vi "Begin.vi"(11 "Image Size":T1=enum."160x120") -> (0 "error out":errorcluster)   [LabVIEW 2012]
doc: "Called before other user functions, this VI is expected to open initial I/O refnums, load in file data, and do all program initialization. Notice that the <B>error out</B> terminal is simply used for data flow. Wiring it to other structures or subVIs ensures that this VI runs first."
uses:
  <vilib>/Rock Robotics/WPI/Camera/WPI_CameraImageSize.ctl
  <vilib>/Rock Robotics/SystemInterfaces/DIO/FPGA_DIOPWMChannel.ctl
  <vilib>/Rock Robotics/WPI/Camera/WPI_CameraWhite Balance Values.ctl
  <vilib>/Rock Robotics/WPI/Camera/WPI_CameraExposure Values.ctl
  <vilib>/Rock Robotics/WPI/Camera/WPI_CameraFrameRate.ctl
  <vilib>/Rock Robotics/WPI/DriverStation/WPI_DriverStationRobotMode2.ctl
  <vilib>/Rock Robotics/WPI/Joystick/WPI_JoystickDeviceEnum.ctl
  <vilib>/Rock Robotics/WPI/SafetyOutput/WPI_SafetyOutputConfigMenu.ctl
  <vilib>/Rock Robotics/SystemInterfaces/DIO/FPGA_DIOChannel.ctl
  <vilib>/Rock Robotics/SystemInterfaces/DIO/FPGA_DIORelayChannel.ctl
  <vilib>/Rock Robotics/WPI/Solenoid/WPI_SolenoidChannel.ctl
  <vilib>/Rock Robotics/SystemInterfaces/Typedef/FPGA_TypedefSolenoidModule.ctl
  <vilib>/Rock Robotics/SystemInterfaces/Typedef/FPGA_TypedefDigitalModule.ctl
  <vilib>/Rock Robotics/SystemInterfaces/Typedef/FPGA_TypedefAnalogModuleForGyro.ctl
  <vilib>/Rock Robotics/SystemInterfaces/AI/FPGA_AIGyroChannel.ctl
  <vilib>/Rock Robotics/WPI/RobotDrive/WPI_RobotDriveOpen2MotorWithJaguar.vi
  Robot Global Data.vi
  <vilib>/Rock Robotics/WPI/RobotDrive/WPI_RobotDriveOpen2MotorWithVictor.vi
  <vilib>/Rock Robotics/WPI/Solenoid/WPI_SolenoidOpenDouble.vi
  <vilib>/Rock Robotics/WPI/Compressor/WPI_CompressorGetSetRefNum.vi
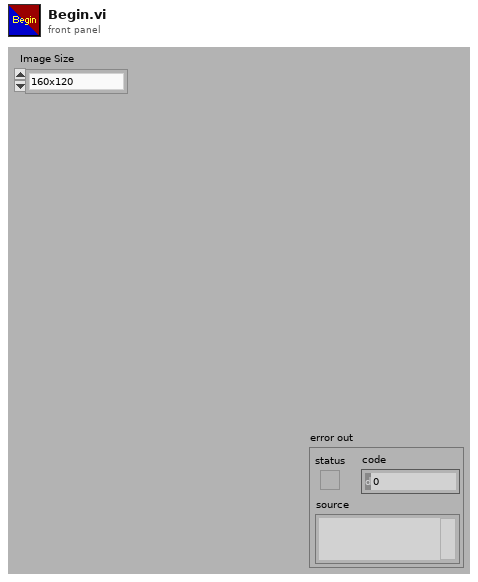
[diagram p1: front panel]
types:
  T1 = typedef "WPI_CameraImageSize.ctl" = enum16{"640x480", "320x240", "160x120"}
  T2 = typedef "FPGA_AIGyroChannel.ctl" = enum8{"AI 1", "AI 2", "Invalid"}
  T3 = typedef "FPGA_TypedefAnalogModuleForGyro.ctl" = enum16{"Analog Module 1"}
  T4 = typedef "FPGA_TypedefDigitalModule.ctl" = enum16{"Digital Module 1", "Digital Module 2"}
  T5 = typedef "WPI_SolenoidChannel.ctl" = enum8{"Solenoid 1", "Solenoid 2", "Solenoid 3", "Solenoid 4", "Solenoid 5", "Solenoid 6", "Solenoid 7", "Solenoid 8", "Invalid"}
  T6 = typedef "FPGA_TypedefSolenoidModule.ctl" = enum16{"Solenoid Module 1", "Solenoid Module 2"}
  T7 = typedef "FPGA_DIORelayChannel.ctl" = enum8{"Relay 1", "Relay 2", "Relay 3", "Relay 4", "Relay 5", "Relay 6", "Relay 7", "Relay 8", "Invalid"}
  T8 = typedef "FPGA_DIOChannel.ctl" = enum8{"DIO 1", "DIO 2", "DIO 3", "DIO 4", "DIO 5", "DIO 6", "DIO 7", "DIO 8", "DIO 9", "DIO 10", "DIO 11", "DIO 12", "DIO 13", "DIO 14", "Invalid"}
  T9 = typedef "WPI_SafetyOutputConfigMenu.ctl" = enum16{"Enable", "Disable"}
  T10 = typedef "FPGA_DIOPWMChannel.ctl" = enum8{"PWM 1", "PWM 2", "PWM 3", "PWM 4", "PWM 5", "PWM 6", "PWM 7", "PWM 8", "PWM 9", "PWM 10", "Invalid"}
  T11 = typedef "WPI_JoystickDeviceEnum.ctl" = enum16{"USB 1", "USB 2", "USB 3", "USB 4", "Kinect 1", "Kinect 2"}
  T12 = typedef "WPI_DriverStationRobotMode2.ctl" = enum16{"Autonomous Disabled", "Autonomous Enabled", "Teleop Disabled", "Teleop Enabled", "Timeout", "Finish", "Test Disabled", "Test Enabled"}
  T13 = typedef "WPI_CameraFrameRate.ctl" = u32
  T14 = typedef "WPI_CameraExposure Values.ctl" = enum16{"Auto", "Flicker-free 50 Hz", "Flicker-free 60 Hz", "Hold current"}
  T15 = typedef "WPI_CameraWhite Balance Values.ctl" = enum16{"Auto", "Fixed indoor", "Fixed outdoor 1", "Fixed outdoor 2", "Fixed fluorescent 1", "Fixed fluorescent 2", "Hold current"}
  T16 = typedef "WPI_CameraDevRef.ctl" = cluster{"Camera Address":string, "CameraStatus":errorcluster, "Acquire Image Notifier":refnum<notifier>}
  T17 = typedef "WPI_JoystickDevRef.ctl" = cluster{"Device":T11}
  T18 = typedef "WPI_RobotDriveDevRef.ctl" = cluster{"DevStatus":errorcluster, "Motors[]":T19[], "Square Inputs":bool, "Max Output":dbl, "Isochronous":bool}
  T19 = typedef "WPI_MotorControlDeviceRef.ctl" = cluster{"DeviceStatus":errorcluster, "Type":enum16{"PWM", "CAN"}, "PWM":cluster{"Digital Module":T4, "PWM Channel":T10, "DeadBand":T20}, "CAN":cluster{"Device Number":u8, "Control Mode":T21, "Semaphore":T22, "Max Vout":dbl}, "Invert":bool, "TransformRef":T23, "InvTransformRef":T23}
  T20 = typedef "WPI_PWMDeadband.ctl" = cluster{"Name":string, "maxPositivePwm":i32, "minPositivePwm":i32, "centerPwm":i32, "maxNegativePwm":i32, "minNegativePwm":i32, "angularRange":u16}
  T21 = typedef "WPI_CANJaguar_ControlMode.ctl" = enum8{"Percent VBus", "Current", "Speed", "Position", "Voltage"}
  T22 = typedef "Semaphore RefNum" = refnum<k1>
  T23 = typedef "WPI_PWMTransform_ConPane.ctl" = refnum<vi>
  T24 = typedef "WPI_CompressorDevRef.ctl" = cluster{"DevStatus":errorcluster, "DigitalInputDevRef":T25, "RelayDevRef":T26}
  T25 = typedef "WPI_DigitalInputDevRef.ctl" = cluster{"DevStatus":errorcluster, "DIO Channel":T8, "Digital Module":T4}
  T26 = typedef "WPI_RelayDevRef.ctl" = cluster{"DevStatus":errorcluster, "Relay Channel":T7, "Digital Module":T4, "Relay Direction":T27}
  T27 = typedef "WPI_RelayDirection.ctl" = enum16{"Both directions", "Forward only", "Reverse only"}
  T28 = typedef "WPI_SolenoidDevRef.ctl" = cluster{"DevStatus":errorcluster, "Solenoid Module":T6, "Forward Solenoid Channel":T5, "Reverse Solenoid Channel":T5}
  T29 = typedef "WPI_GyroDevRef.ctl" = cluster{"DevStatus":errorcluster, "Analog Module":T30, "Analog Channel":T31, "Offset":dbl, "Gain (VoltsPerDegree/Second)":dbl}
  T30 = typedef "FPGA_TypedefAnalogModule.ctl" = enum16{"Analog Module 1", "Analog Module 2"}
  T31 = typedef "FPGA_AIChannel.ctl" = enum8{"AI 1", "AI 2", "AI 3", "AI 4", "AI 5", "AI 6", "AI 7", "AI 8", "Invalid"}
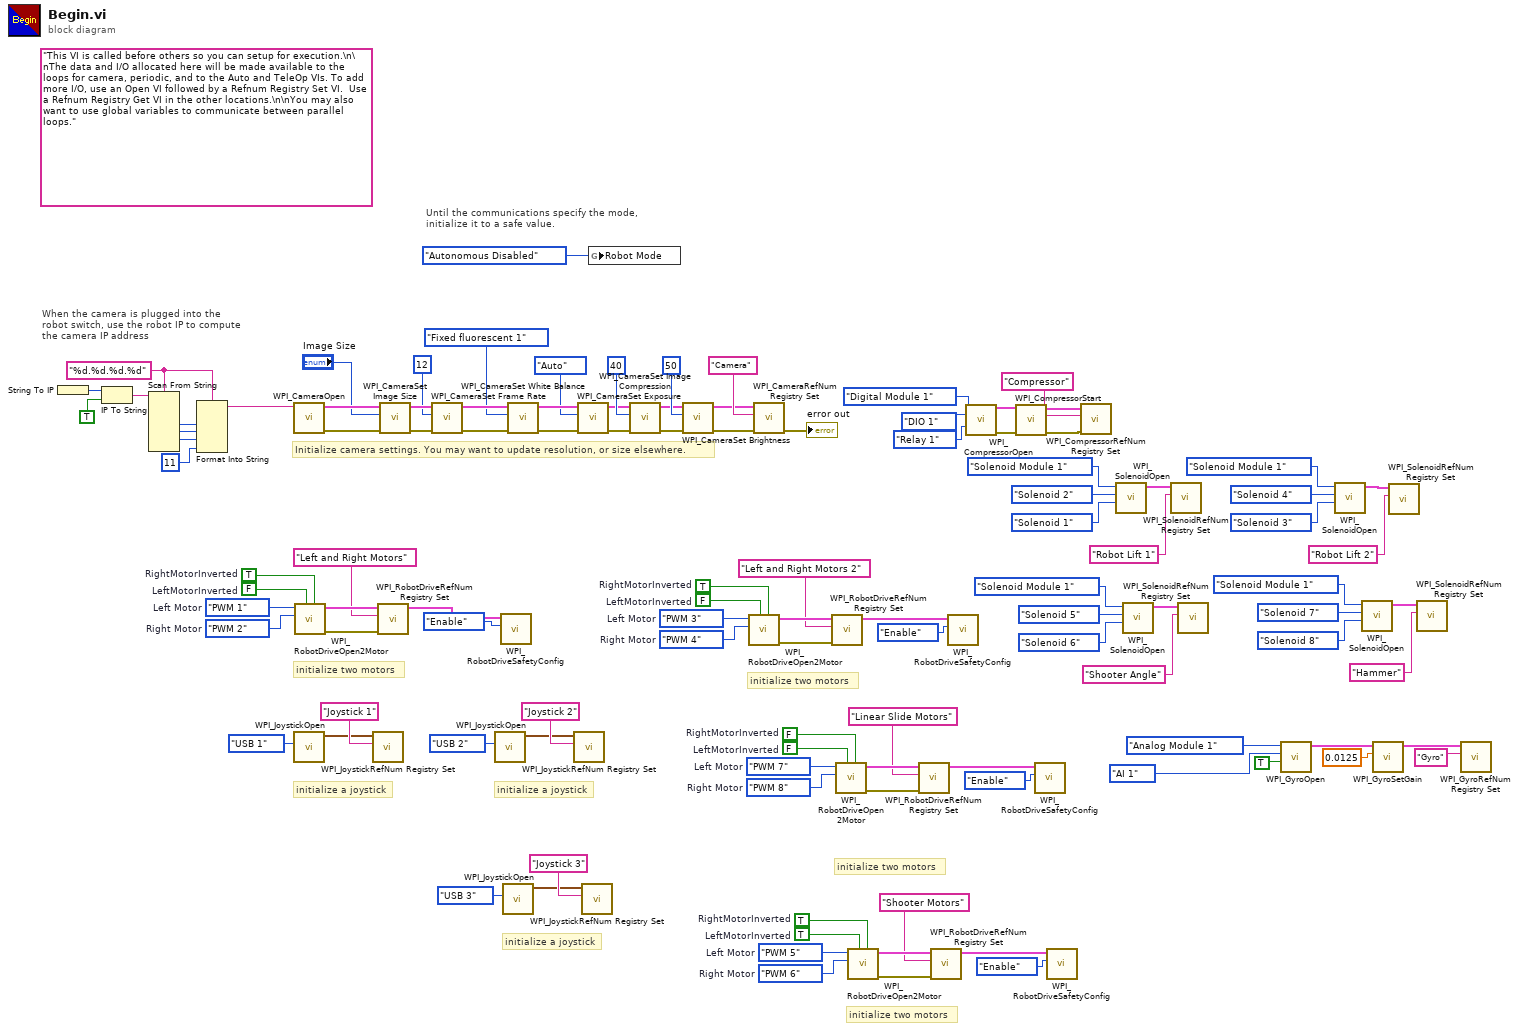
[diagram p0: block diagram]
diagram:
  w38 = FPGA_DIOPWMChannel."PWM 6"  # Right Motor
  w39 = FPGA_DIOPWMChannel."PWM 5"  # Left Motor
  w43 = TRUE  # LeftMotorInverted
  w44 = TRUE  # RightMotorInverted
  w50 = FPGA_DIOPWMChannel."PWM 8"  # Right Motor
  w51 = FPGA_DIOPWMChannel."PWM 7"  # Left Motor
  w55 = FALSE  # LeftMotorInverted
  w56 = FALSE  # RightMotorInverted
  w59 = FPGA_DIOPWMChannel."PWM 4"  # Right Motor
  w60 = FPGA_DIOPWMChannel."PWM 3"  # Left Motor
  w64 = FALSE  # LeftMotorInverted
  w65 = TRUE  # RightMotorInverted
  w77 = "%d.%d.%d.%d" ("format string")
  (unwired) "This VI is called before others so you can setup for execution.\n\nThe data and I/O allocated here will be made available to the loops for camera, periodic, and to the Auto and TeleOp VIs. To add more I/O, use an Open VI followed by a Refnum Registry Set VI.  Use a Refnum Registry Get VI in the other locations.\n\nYou may also want to use global variables to communicate between parallel loops."
  w88 = FPGA_DIOPWMChannel."PWM 2"  # Right Motor
  w89 = FPGA_DIOPWMChannel."PWM 1"  # Left Motor
  w111 = FALSE  # LeftMotorInverted
  w112 = TRUE  # RightMotorInverted
  # "initialize two motors"
  # "initialize a joystick"
  # "initialize two motors"
  # "initialize two motors"
  # "initialize a joystick"
  # "initialize a joystick"
  # "Until the communications specify the mode,\ninitialize it to a safe value."
  # "When the camera is plugged into the\nrobot switch, use the robot IP to compute\nthe camera IP address"
  # "initialize two motors"
  # "Initialize camera settings. You may want to update resolution, or size elsewhere."
  n1 = String To IP() -> (0:w84:u32)  [unwired: 1 in]
  n2 = IP To String(1:TRUE ("dot notation? (F)"), 2:w84) -> (0:w82:string)
  n3 = Scan From String(format string=w77, input string=w82) -> (output 1=w81:i32, output 2=w80:i32, output 3=w79:i32)  [unwired: 7 in, 3 out]
  n4 = Format Into String(format string=w77, w81, w80, w79, 11 ("Compression")) -> (resulting string=w73:string)  [unwired: 2 in, 1 out]
  n5 = call <vilib>:"WPI_CameraOpen.vi"("Camera Address"=w73) -> ("error out"=w98:errorcluster, "CameraDevRef"=w99:T16)  [unwired: 1 in, 8 out]
  n6 = call <vilib>:"WPI_JoystickOpen.vi"("JoystickDevice"=WPI_JoystickDeviceEnum."USB 1") -> ("JoystickDevRef"=w71:T17)  [unwired: 10 in]
  n7 = call-poly <vilib>:"WPI_RobotDriveOpen2Motor.vi"("Right Motor Inverted"=w112, "Left Motor Inverted"=w111, "Right Motor"=w88, "Left Motor"=w89) -> ("error out"=w107:errorcluster, "RobotDriveDevRef"=w109:T18)  [unwired: 1 in, 5 out]
  n8 = call <vilib>:"WPI_JoystickRefNum Registry Set.vi"("refnum name"="Joystick 1", "JoystickDevRef"=w71) -> ()  [unwired: 8 in, 2 out]
  n9 = call <vilib>:"WPI_RobotDriveRefNum Registry Set.vi"("error in (no error)"=w107, "refnum name"="Left and Right Motors", "RobotDriveDevRef"=w109) -> ("RobotDriveDevRef"=w76:T18)  [unwired: 8 out]
  n10 = call <vilib>:"WPI_CameraSet Image Size.vi"("error in (no error)"=w98, "Image Size"="Image Size", "CameraDevRef"=w99) -> ("error out"=w97:errorcluster, "CameraDevRef Out"=w100:T16)  [unwired: 7 out]
  n11 = call <vilib>:"WPI_CameraSet Frame Rate.vi"("error in (no error)"=w97, "Frame Rate (fps)"=T13 12, "CameraDevRef"=w100) -> ("error out"=w96:errorcluster, "CameraDevRef Out"=w102:T16)  [unwired: 7 out]
  n12 = call <vilib>:"WPI_JoystickOpen.vi"("JoystickDevice"=WPI_JoystickDeviceEnum."USB 2") -> ("JoystickDevRef"=w67:T17)  [unwired: 10 in]
  n13 = call <vilib>:"WPI_RobotDriveSafetyConfig.vi"("mode"=WPI_SafetyOutputConfigMenu."Enable", "RobotDriveDevRef"=w76) -> ()  [unwired: 8 in, 2 out]
  n14 = call <vilib>:"WPI_JoystickOpen.vi"("JoystickDevice"=WPI_JoystickDeviceEnum."USB 3") -> ("JoystickDevRef"=w46:T17)  [unwired: 10 in]
  n15 = call <vilib>:"WPI_CameraSet White Balance.vi"("error in (no error)"=w96, "White Balance"=WPI_CameraWhite_Balance_Values."Fixed fluorescent 1", "CameraDevRef"=w102) -> ("error out"=w95:errorcluster, "CameraDevRef Out"=w101:T16)  [unwired: 7 out]
  n16 = call <vilib>:"WPI_JoystickRefNum Registry Set.vi"("refnum name"="Joystick 2", "JoystickDevRef"=w67) -> ()  [unwired: 8 in, 2 out]
  n17 = call <vilib>:"WPI_CameraSet Exposure.vi"("error in (no error)"=w95, "Exposure"=WPI_CameraExposure_Values."Auto", "CameraDevRef"=w101) -> ("error out"=w94:errorcluster, "CameraDevRef Out"=w104:T16)  [unwired: 7 out]
  n18 = call <vilib>:"WPI_JoystickRefNum Registry Set.vi"("refnum name"="Joystick 3", "JoystickDevRef"=w46) -> ()  [unwired: 8 in, 2 out]
  n19 = global write "Robot Global Data.vi" "Robot Mode"(WPI_DriverStationRobotMode2."Autonomous Disabled" ("Robot Mode")) -> ()
  n20 = call <vilib>:"WPI_CameraSet Image Compression.vi"("error in (no error)"=w94, "Compression"=40, "CameraDevRef"=w104) -> ("error out"=w93:errorcluster, "CameraDevRef Out"=w103:T16)  [unwired: 7 out]
  n21 = call <vilib>:"WPI_CameraSet Brightness.vi"("error in (no error)"=w93, "Brightness"=50, "CameraDevRef"=w103) -> ("error out"=w91:errorcluster, "CameraDevRef Out"=w92:T16)  [unwired: 7 out]
  n22 = call-poly <vilib>:"WPI_RobotDriveOpen2Motor.vi"("Right Motor Inverted"=w65, "Left Motor Inverted"=w64, "Right Motor"=w59, "Left Motor"=w60) -> ("error out"=w61:errorcluster, "RobotDriveDevRef"=w63:T18)  [unwired: 1 in, 5 out]
  n23 = call <vilib>:"WPI_CameraRefNum Registry Set.vi"("error in (no error)"=w91, "refnum name"="Camera", "CameraDevRef"=w92) -> ("error out"=→"error out":errorcluster)  [unwired: 8 out]
  n24 = call <vilib>:"WPI_RobotDriveRefNum Registry Set.vi"("error in (no error)"=w61, "refnum name"="Left and Right Motors 2", "RobotDriveDevRef"=w63) -> ("RobotDriveDevRef"=w58:T18)  [unwired: 8 out]
  n25 = call-poly <vilib>:"WPI_RobotDriveOpen2Motor.vi"("Right Motor Inverted"=w56, "Left Motor Inverted"=w55, "Right Motor"=w50, "Left Motor"=w51) -> ("error out"=w52:errorcluster, "RobotDriveDevRef"=w54:T18)  [unwired: 1 in, 5 out]
  n26 = call-poly <vilib>:"WPI_RobotDriveOpen2Motor.vi"("Right Motor Inverted"=w44, "Left Motor Inverted"=w43, "Right Motor"=w38, "Left Motor"=w39) -> ("error out"=w40:errorcluster, "RobotDriveDevRef"=w42:T18)  [unwired: 1 in, 5 out]
  n27 = call <vilib>:"WPI_RobotDriveRefNum Registry Set.vi"("error in (no error)"=w52, "refnum name"="Linear Slide Motors", "RobotDriveDevRef"=w54) -> ("RobotDriveDevRef"=w49:T18)  [unwired: 8 out]
  n28 = call <vilib>:"WPI_RobotDriveRefNum Registry Set.vi"("error in (no error)"=w40, "refnum name"="Shooter Motors", "RobotDriveDevRef"=w42) -> ("RobotDriveDevRef"=w37:T18)  [unwired: 8 out]
  n29 = call <vilib>:"WPI_RobotDriveSafetyConfig.vi"("mode"=WPI_SafetyOutputConfigMenu."Enable", "RobotDriveDevRef"=w58) -> ()  [unwired: 8 in, 2 out]
  n30 = call <vilib>:"WPI_CompressorOpen.vi"("Pressure Switch Digital Module (Module 1)"=FPGA_TypedefDigitalModule."Digital Module 1", "Pressure Switch DIO Channel"=FPGA_DIOChannel."DIO 1", "Relay Channel"=FPGA_DIORelayChannel."Relay 1") -> ("CompressorDevRef"=w35:T24, "error out"=w10:errorcluster)  [unwired: 2 in, 9 out]
  n31 = call <vilib>:"WPI_CompressorStart.vi"("error in (no error)"=w10, "CompressorDevRef"=w35) -> ("error out"=w9:errorcluster, "CompressorDevRef"=w32:T24)  [unwired: 8 out]
  n32 = call <vilib>:"WPI_RobotDriveSafetyConfig.vi"("mode"=WPI_SafetyOutputConfigMenu."Enable", "RobotDriveDevRef"=w49) -> ()  [unwired: 8 in, 2 out]
  n33 = call <vilib>:"WPI_RobotDriveSafetyConfig.vi"("mode"=WPI_SafetyOutputConfigMenu."Enable", "RobotDriveDevRef"=w37) -> ()  [unwired: 8 in, 2 out]
  n34 = call <vilib>:"WPI_CompressorRefNum Registry Set.vi"("error in (no error)"=w9, "refnum name"="Compressor", "CompressorDevRef"=w32) -> ()  [unwired: 7 in, 2 out]
  n35 = call-poly <vilib>:"WPI_SolenoidOpen.vi"("Reverse Solenoid Channel"=WPI_SolenoidChannel."Solenoid 1", "Forward Solenoid Channel"=WPI_SolenoidChannel."Solenoid 2" ("Solenoid Channel"), "Solenoid Module (Module 1)"=FPGA_TypedefSolenoidModule."Solenoid Module 1") -> ("SolenoidDevRef"=w30:T28)  [unwired: 7 in, 1 out]
  n36 = call-poly <vilib>:"WPI_SolenoidOpen.vi"("Reverse Solenoid Channel"=WPI_SolenoidChannel."Solenoid 6", "Forward Solenoid Channel"=WPI_SolenoidChannel."Solenoid 5" ("Solenoid Channel"), "Solenoid Module (Module 1)"=FPGA_TypedefSolenoidModule."Solenoid Module 1") -> ("SolenoidDevRef"=w17:T28)  [unwired: 7 in, 1 out]
  n37 = call <vilib>:"WPI_SolenoidRefNum Registry Set.vi"("refnum name"="Robot Lift 1", "SolenoidDevRef"=w30) -> ()  [unwired: 8 in, 2 out]
  n38 = call <vilib>:"WPI_SolenoidRefNum Registry Set.vi"("refnum name"="Shooter Angle", "SolenoidDevRef"=w17) -> ()  [unwired: 8 in, 2 out]
  n39 = call <vilib>:"WPI_GyroOpen.vi"("Calibrate On Open"=TRUE, "Analog Channel"=FPGA_AIGyroChannel."AI 1", "Analog Module (Module 1)"=FPGA_TypedefAnalogModuleForGyro."Analog Module 1") -> ("GyroDevRef"=w3:T29)  [unwired: 6 in, 2 out]
  n40 = call-poly <vilib>:"WPI_SolenoidOpen.vi"("Reverse Solenoid Channel"=WPI_SolenoidChannel."Solenoid 3", "Forward Solenoid Channel"=WPI_SolenoidChannel."Solenoid 4" ("Solenoid Channel"), "Solenoid Module (Module 1)"=FPGA_TypedefSolenoidModule."Solenoid Module 1") -> ("SolenoidDevRef"=w26:T28)  [unwired: 7 in, 1 out]
  n41 = call-poly <vilib>:"WPI_SolenoidOpen.vi"("Reverse Solenoid Channel"=WPI_SolenoidChannel."Solenoid 8", "Forward Solenoid Channel"=WPI_SolenoidChannel."Solenoid 7" ("Solenoid Channel"), "Solenoid Module (Module 1)"=FPGA_TypedefSolenoidModule."Solenoid Module 1") -> ("SolenoidDevRef"=w16:T28)  [unwired: 7 in, 1 out]
  n42 = call <vilib>:"WPI_GyroSetGain.vi"("Gain (VoltsPerDegree/Second)"=0.0125, "GyroDevRef"=w3) -> ("GyroDevRef"=w2:T29)  [unwired: 8 in, 1 out]
  n43 = call <vilib>:"WPI_SolenoidRefNum Registry Set.vi"("refnum name"="Robot Lift 2", "SolenoidDevRef"=w26) -> ()  [unwired: 8 in, 2 out]
  n44 = call <vilib>:"WPI_SolenoidRefNum Registry Set.vi"("refnum name"="Hammer", "SolenoidDevRef"=w16) -> ()  [unwired: 8 in, 2 out]
  n45 = call <vilib>:"WPI_GyroRefNum Registry Set.vi"("refnum name"="Gyro", "GyroDevRef"=w2) -> ()  [unwired: 8 in, 2 out]
